vi "Kalman filter.vi"(1 "New data":T1, 2 "Reset":bool, 3 "Constants":T2={"Q_Angle"=0.001, "Q_Bias"=0.003, "R_measure"=0.03}) -> (0 "Angle out":dbl)   [LabVIEW 2013]
panel:
  # "Kalman filter"
  # "https://github.com/TKJElectronics/KalmanFilter/blob/master/Kalman.h"
  # "New angle from\naccelerometer\nin degrees"
  # "New rate from gyroscope in degrees per second"
  # "Time constant"
  # "Process noise variance\nfor the accelerometer"
  # "Process noise variance\nfor the gyro bias"
  # "Measurement noise variance - \nthis is actually the variance \nof the measurement noise"
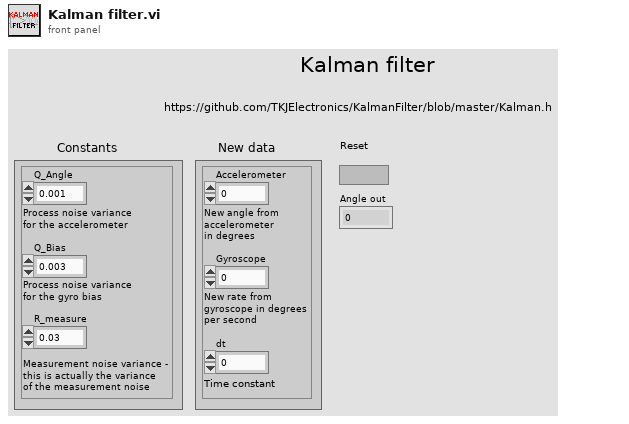
[diagram p1: front panel]
types:
  T1 = cluster{"Accelerometer":dbl, "Gyroscope":dbl, "dt":dbl}
  T2 = cluster{"Q_Angle":dbl, "Q_Bias":dbl, "R_measure":dbl}
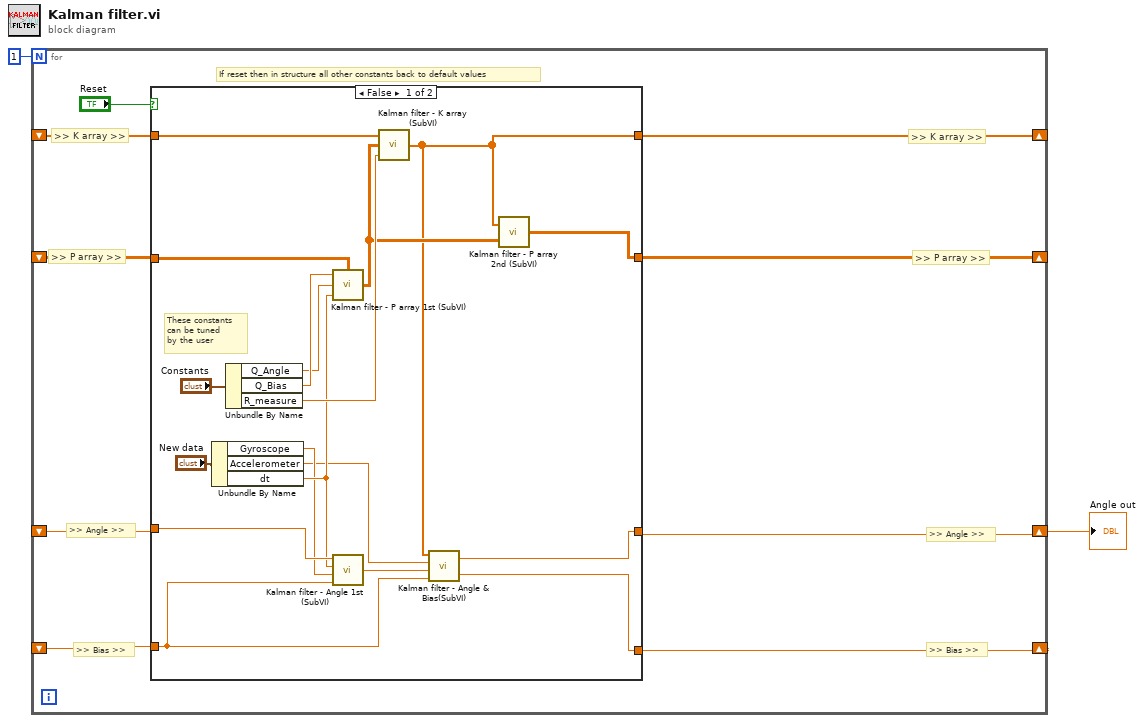
[diagram p0: block diagram]
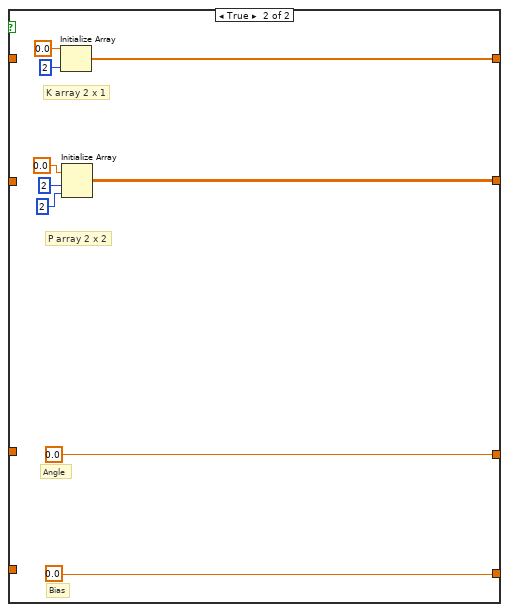
[diagram p2: hidden frame]
diagram:
  n1 = for {
    N: 1 -> [_]
    shift-right: [w10] -> w1
    shift-left: _ -> [w11]
    shift-right: [w8] -> _
    shift-left: _ -> [w7]
    shift-right: [w6] -> _
    shift-left: _ -> [w5]
    shift-right: [w4] -> _
    shift-left: _ -> [w3]
    # ">> P array >>"
    # ">> P array >>"
    # ">> K array >>"
    # ">> K array >>"
    # ">> Bias >>"
    # ">> Angle >>"
    # ">> Bias >>"
    # ">> Angle >>"
    # "If reset then in structure all other constants back to default values"
    n2 = case shown="False" "Reset" {
      tunnel: w11 -> [w23 _]
      tunnel: [w13 0.0] -> w10
      tunnel: [w12 0.0] -> w8
      tunnel: w7 -> [w18 _]
      tunnel: [w15 w33] -> w6
      tunnel: w5 -> [w17 _]
      tunnel: [w14 w30] -> w4
      tunnel: w3 -> [w24 _]
      frame False {
        # "These constants\ncan be tuned\nby the user"
        n3 = Unbundle By Name("New data") -> ("Gyroscope"=w21:dbl, "Accelerometer"=w20:dbl, "dt"=w22:dbl)
        n4 = Unbundle By Name("Constants") -> ("Q_Angle"=w26:dbl, "Q_Bias"=w27:dbl, "R_measure"=w25:dbl)
        n5 = call "Kalman filter - P array 1st (SubVI).vi"("P Array In"=w17, "dt"=w22, "Q_Angle"=w26, "Q_Bias"=w27) -> ("P Array out"=w16:dbl[][])
        n6 = call "Kalman filter - Angle 1st (SubVI).vi"("Bias"=w18, "Gyroscope"=w21, "dt"=w22, "Angle in"=w23) -> ("Angle out"=w19:dbl)
        n7 = call "Kalman filter - K array (SubVI).vi"("R_measure"=w25, "P Array in"=w16, "K Array in"=w24) -> ("K Array out"=w14:dbl[])
        n8 = call "Kalman filter - Angle & Bias(SubVI).vi"("Bias in"=w18, "Angle in"=w19, "Accelerometer"=w20, "K Array in"=w14) -> ("Bias out"=w12:dbl, "Angle out"=w13:dbl)
        n9 = call "Kalman filter - P array 2nd (SubVI).vi"("P Array in"=w16, "K Array in"=w14) -> ("P Array out"=w15:dbl[][])
      }
      frame True {
        # "K array 2 x 1"
        # "P array 2 x 2"
        # "Bias"
        # "Angle"
        n10 = Initialize Array(0.0 ("element"), 2 ("dimension size")) -> (w30:dbl[])
        n11 = Initialize Array(0.0 ("element"), 2 ("dimension size"), 2 ("dimension size")) -> (w33:dbl[][])
      }
    }
  }
  "Angle out" <- w1
